vi "Global 1.vi"() -> ()   [LabVIEW 2019]
uses:
  <userlib>/KNR OS 4.2 LabVIEW Toolkit/Type Definition/KNR3 Reference.ctl
  <userlib>/_FPGA Interface Advanced Tools/FPGA Interface Base/FPGA Interface Base.lvclass
  <userlib>/KNR OS 4.2 LabVIEW Toolkit/Type Definition/Resource.ctl
panel:
  in  "re":dbl=194.88 format="%#_13g"
  in  "e":dbl=39.092 format="%#_13g"
  in  "f":dbl=63.127 format="%#_13g"
  in  "rf":dbl=125.28 format="%#_13g"
  in  "調機參數":T1={"等比調整到角度正確"={"S1"=1.18, "S2"=1.18, "S3"=1.2, "S4"=5.73, "S5"=0.68}, "補償角度到0度是水平"={"S1"=0.0, "S2"=0.0, "S3"=0.0, "S4"=400.0, "S5"=135.0}}
  in  "origin?":bool
  in  "z":dbl(slide) scale=-135.0..50.0
  in  "y":dbl(slide) scale=-115.0..115.0
  in  "x":dbl(slide) scale=-115.0..115.0
  out "KNR3 Reference":T2
  in  "RC Pulse Width (1500 uS)":u16[](array[numeric])=[1500, 1500, 1500, 1500, 1500, 1500, 1500]
  out "thetaZ":dbl
  out "thetaY":dbl
  out "thetaX":dbl
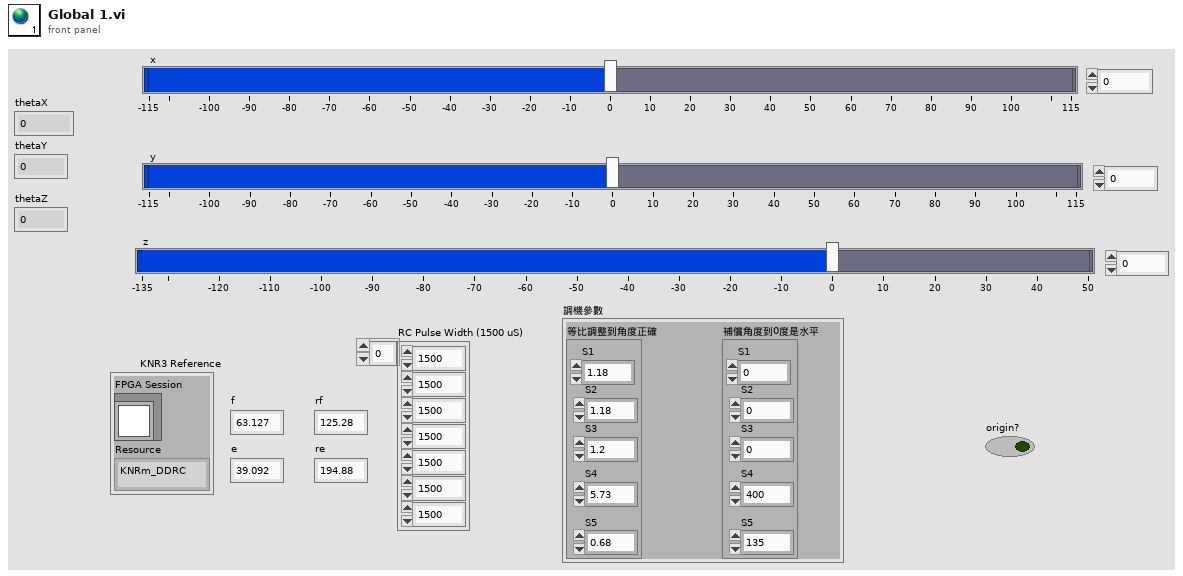
[diagram p1: front panel]
types:
  T1 = cluster{"等比調整到角度正確":cluster{"S1":dbl, "S2":dbl, "S3":dbl, "S4":dbl, "S5":dbl}, "補償角度到0度是水平":cluster{"S1":dbl, "S2":dbl, "S3":dbl, "S4":dbl, "S5":dbl}}
  T2 = typedef "KNR3 Reference.ctl" = cluster{"FPGA Session":refnum<class "FPGA Interface Base.lvclass">, "Resource":T3}
  T3 = typedef "Resource.ctl" = enum16{"KNRm_DDRC", "KNRm_DDDD", "KNRm_DDDR", "KNRm_DDDC", "KNR", "KNRm_neww"}
diagram:
